vi "StoreDefaultParams.vi"(8 "error in (no error)":errorcluster, 10 "DefaultINIParams":T1={"Handle"="", "eFunction"=0, "dRange"=0.0, "dResolution"=0.0, "eTriggerSource"=0, "dTriggerDelay"=0.0, "iMaxTimeMilliseconds"=0, "eMeasCompleteDest"=0, "iTriggerCount"=0, "iSampleCount"=0, "eSampleClock"=0, "dSampleInterval"=0.0, "iMaxTimeMillisecondsMultiPoint"=0, "iArraySize"=0, "dMinFreq"=0.0, "dMaxFreq"=0.0, "dFrequencyVoltageRange"=0.0, "eEdge"=10280, "sSource"="", "eEdgeSample"=10280, "sSourceSample"=""} {"eEdgeSample" items=["Rising"=10280, "Falling"=10171]; "eEdge" items=["Rising"=10280, "Falling"=10171]; "eSampleClock" items=["NULL"=0, "Immediate"=1, "External"=2, "Software Trigger"=3, "Interval"=10]; "eMeasCompleteDest" items=["None"=0, "External"=2]; "eTriggerSource" items=["NULL", "Immediate", "External", "Software Trigger"]; "eFunction" items=["NULL"=0, "DC Volts"=1, "AC Volts"=2, "DC Current"=3, "AC Current"=4, "Frequency"=104, "AC Coupled Direct Sampling"=1005]}, 11 "NISTSamplerPluginsBase in":refnum<class "SamplerPluginsBase.lvclass">) -> (0 "error out":errorcluster, 3 "NISTSamplerPluginsBase out":refnum<class "SamplerPluginsBase.lvclass">)   [LabVIEW 2014, in "SamplerPlugins.lvlib" / "SamplerPluginsBase.lvclass"]
uses:
  SamplerPluginsBase.lvclass
  TypeDefs/ConfigMultiPointParams.ctl
  TypeDefs/MultiPointParams.ctl
  TypeDefs/ConfigACBandwidthParams.ctl
  TypeDefs/TriggerParams.ctl
  TypeDefs/DefaultINIParams.ctl
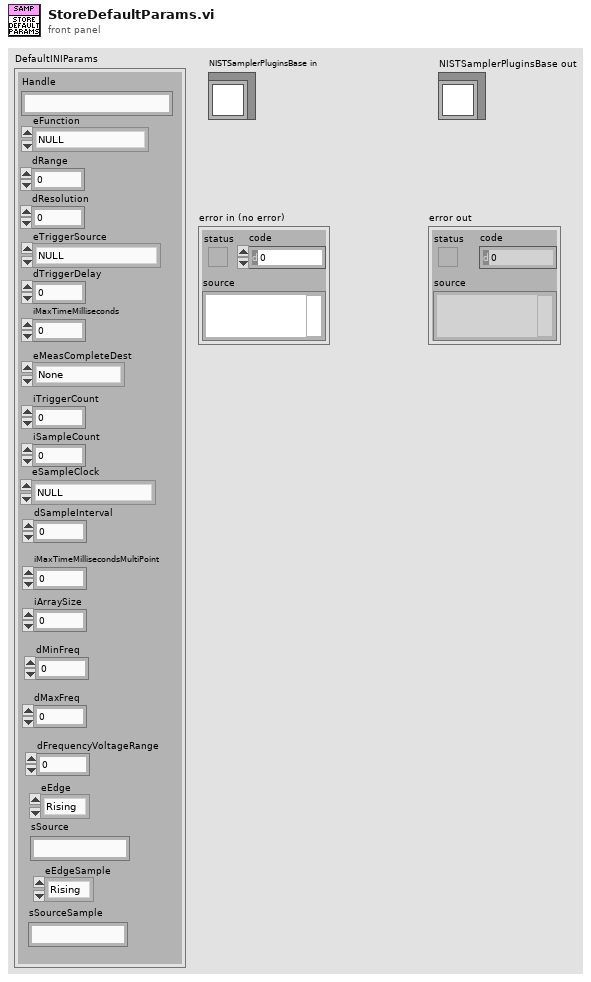
[diagram p1: front panel]
types:
  T1 = typedef "SamplerPlugins.lvlib/SamplerPluginsBase.lvclass/DefaultINIParams.ctl" = cluster{"Handle":string, "eFunction":u16, "dRange":dbl, "dResolution":dbl, "eTriggerSource":u16, "dTriggerDelay":dbl, "iMaxTimeMilliseconds":i32, "eMeasCompleteDest":u16, "iTriggerCount":i32, "iSampleCount":i32, "eSampleClock":u16, "dSampleInterval":dbl, "iMaxTimeMillisecondsMultiPoint":i32, "iArraySize":i32, "dMinFreq":dbl, "dMaxFreq":dbl, "dFrequencyVoltageRange":dbl, "eEdge":u16, "sSource":string, "eEdgeSample":u16, "sSourceSample":string}
  T2 = typedef "SamplerPlugins.lvlib/SamplerPluginsBase.lvclass/TriggerParams.ctl" = cluster{"eEdge":u16, "sSource":string}
  T3 = typedef "SamplerPlugins.lvlib/SamplerPluginsBase.lvclass/ConfigACBandwidthParams.ctl" = cluster{"dMinFreq":dbl, "dMaxFreq":dbl}
  T4 = typedef "SamplerPlugins.lvlib/SamplerPluginsBase.lvclass/MultiPointParams.ctl" = cluster{"iMaxTimeMilliseconds":i32, "iArraySize":i32}
  T5 = typedef "SamplerPlugins.lvlib/SamplerPluginsBase.lvclass/ConfigMultiPointParams.ctl" = cluster{"iTriggerCount":i32, "iSampleCount":i32, "eSampleClock":u16, "dSampleInterval":dbl}
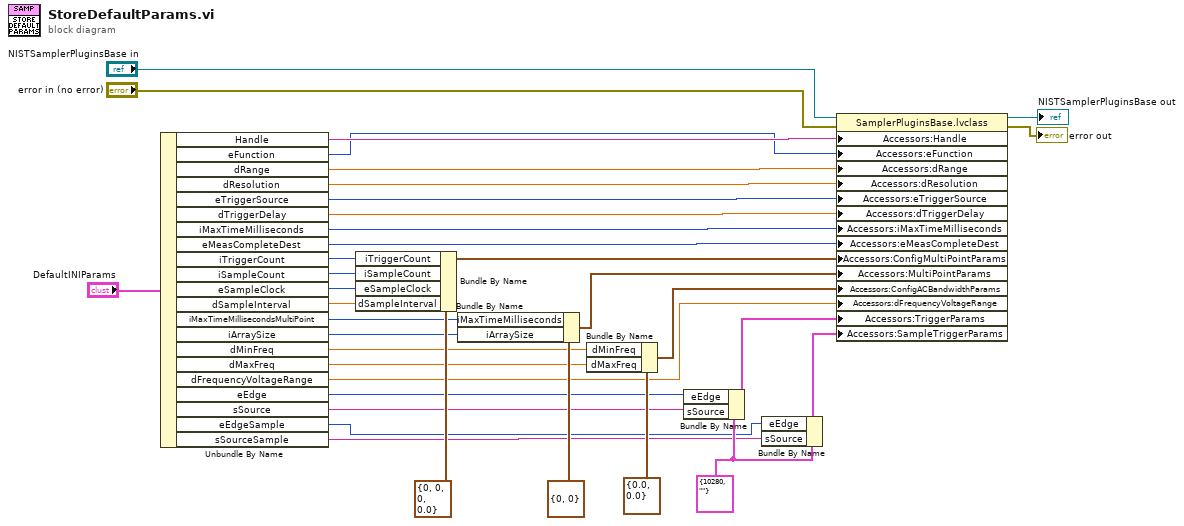
[diagram p0: block diagram]
diagram:
  w5 = T2 {"eEdge"=10280, "sSource"=""} ("TriggerParams")
  n1 = Unbundle By Name("DefaultINIParams") -> ("Handle"=w30:string, "eFunction"=w29:u16, "dRange"=w28:dbl, "dResolution"=w27:dbl, "eTriggerSource"=w26:u16, "dTriggerDelay"=w25:dbl, "iMaxTimeMilliseconds"=w24:i32, "eMeasCompleteDest"=w23:u16, "iTriggerCount"=w21:i32, "iSampleCount"=w20:i32, "eSampleClock"=w19:u16, "dSampleInterval"=w18:dbl, "iMaxTimeMillisecondsMultiPoint"=w15:i32, "iArraySize"=w14:i32, "dMinFreq"=w11:dbl, "dMaxFreq"=w10:dbl, "dFrequencyVoltageRange"=w9:dbl, "eEdge"=w7:u16, "sSource"=w6:string, "eEdgeSample"=w2:u16, "sSourceSample"=w1:string)
  n2 = Bundle By Name(cluster=T5 {"iTriggerCount"=0, "iSampleCount"=0, "eSampleClock"=0, "dSampleInterval"=0.0} ("ConfigMultiPointParams"), "iTriggerCount"=w21, "iSampleCount"=w20, "eSampleClock"=w19, "dSampleInterval"=w18) -> (w17:T5)
  n3 = Bundle By Name(cluster=T4 {"iMaxTimeMilliseconds"=0, "iArraySize"=0} ("ReadMultiPointParams"), "iMaxTimeMilliseconds"=w15, "iArraySize"=w14) -> (w13:T4)
  n4 = Bundle By Name(cluster=T3 {"dMinFreq"=0.0, "dMaxFreq"=0.0} ("ConfigACBandwidthParams"), "dMinFreq"=w11, "dMaxFreq"=w10) -> (w3:T3)
  n5 = Bundle By Name(cluster=w5, "eEdge"=w7, "sSource"=w6) -> (w8:T2)
  n6 = Bundle By Name(cluster=w5, "eEdge"=w2, "sSource"=w1) -> (w4:T2)
  n7 = property class="SamplerPluginsBase.lvclass"(reference="NISTSamplerPluginsBase in", error in="error in (no error)", "Accessors:Handle"=w30, "Accessors:eFunction"=w29, "Accessors:dRange"=w28, "Accessors:dResolution"=w27, "Accessors:eTriggerSource"=w26, "Accessors:dTriggerDelay"=w25, "Accessors:iMaxTimeMilliseconds"=w24, "Accessors:eMeasCompleteDest"=w23, "Accessors:ConfigMultiPointParams"=w17, "Accessors:MultiPointParams"=w13, "Accessors:ConfigACBandwidthParams"=w3, "Accessors:dFrequencyVoltageRange"=w9, "Accessors:TriggerParams"=w8, "Accessors:SampleTriggerParams"=w4) -> (reference out=→"NISTSamplerPluginsBase out":refnum<class "SamplerPluginsBase.lvclass">, error out=→"error out":errorcluster)
